vi "CalculateOffsets.vi"(4 "Dynamic LF":dbl, 5 "Static LF":dbl, 6 "GF":dbl) -> (0 "Dynamic LF Offset":dbl, 1 "Static LF Offset":dbl, 2 "GF Offset":dbl)   [LabVIEW 2020]
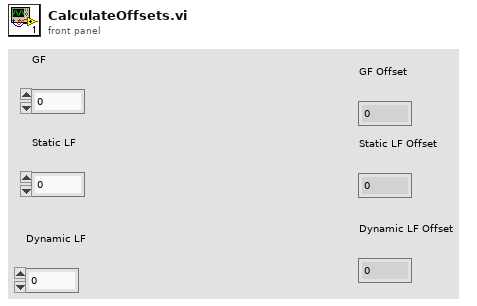
[diagram p1: front panel]
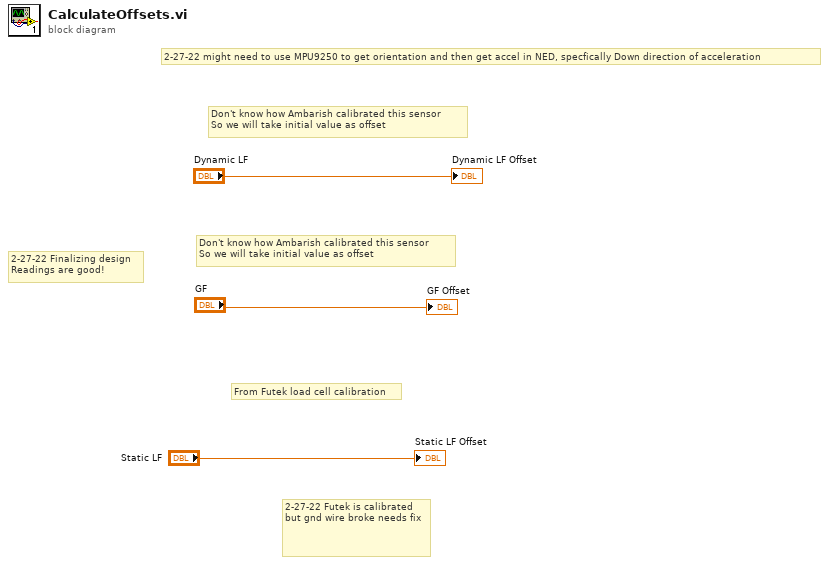
[diagram p0: block diagram]
diagram:
  # "2-27-22 might need to use MPU9250 to get orientation and then get accel in NED, specfically Down direction of acceleration"
  # "2-27-22 Futek is calibrated\nbut gnd wire broke needs fix"
  # "2-27-22 Finalizing design\nReadings are good!"
  # "Don't know how Ambarish calibrated this sensor\nSo we will take initial value as offset"
  # "Don't know how Ambarish calibrated this sensor\nSo we will take initial value as offset"
  # "From Futek load cell calibration"
  "Static LF Offset" <- "Static LF"
  "Dynamic LF Offset" <- "Dynamic LF"
  "GF Offset" <- "GF"
